vi "PC Op Mode Translate.vi"(3 "Op Mode In":u16) -> (1 "Op Mode Out":T1)   [LabVIEW 2014]
uses:
  Controls/MicroZed Config Op Mode.ctl
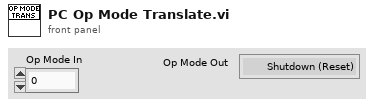
[diagram p1: front panel]
types:
  T1 = typedef "MicroZed Config Op Mode.ctl" = enum16{"Shutdown (Reset)", "Startup", "Idle", "Voltage Mode", "Current Mode", "Fault", "OL Voltage (Debug)", "No Data"}
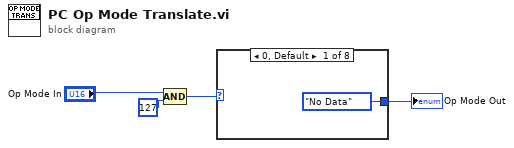
[diagram p0: block diagram]
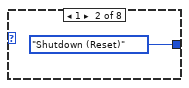
[diagram p2: hidden frame]
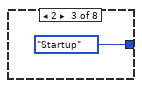
[diagram p3: hidden frame]
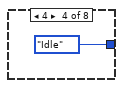
[diagram p4: hidden frame]
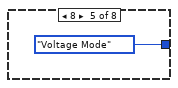
[diagram p5: hidden frame]
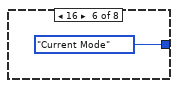
[diagram p6: hidden frame]
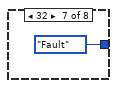
[diagram p7: hidden frame]
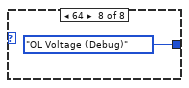
[diagram p8: hidden frame]
diagram:
  n1 = Compound Arithmetic op=AND("Op Mode In", u16 127 ("value")) -> (w2:u16)
  n2 = case shown="0, Default" w2 {
    tunnel: [MicroZed_Config_Op_Mode."No Data" ("Op Mode Out") MicroZed_Config_Op_Mode."Shutdown (Reset)" ("Op Mode Out") MicroZed_Config_Op_Mode."Startup" ("Op Mode Out") MicroZed_Config_Op_Mode."Idle" ("Op Mode Out") MicroZed_Config_Op_Mode."Voltage Mode" ("Op Mode Out") MicroZed_Config_Op_Mode."Current Mode" ("Op Mode Out") MicroZed_Config_Op_Mode."Fault" ("Op Mode Out") MicroZed_Config_Op_Mode."OL Voltage (Debug)" ("Op Mode Out")] -> w4
    frame 0, Default {
    }
    frame 1 {
    }
    frame 2 {
    }
    frame 4 {
    }
    frame 8 {
    }
    frame 16 {
    }
    frame 32 {
    }
    frame 64 {
    }
  }
  "Op Mode Out" <- w4
